vi "New.vi"(8 "error in (no error)":errorcluster, 11 "reference in":refnum<class "[Test Suite] File Transfer Helpers.lvclass">) -> (0 "error out":errorcluster, 3 "reference out":refnum<class "[Test Suite] File Transfer Helpers.lvclass">)   [LabVIEW 2015, in "Tests.lvlib" / "[Test Suite] File Transfer Helpers.lvclass"]
uses:
  [Test Suite] File Transfer Helpers.lvclass
  <vilib>/addons/_JKI Toolkits/VI Tester/TestCase.llb/TestCase.lvclass
  [Test Suite] File Transfer Helpers.lvclass/[Test Suite] File Transfer Helpers.ctl
  <vilib>/addons/_JKI Toolkits/VI Tester/TestSuite.llb/TestSuite.lvclass
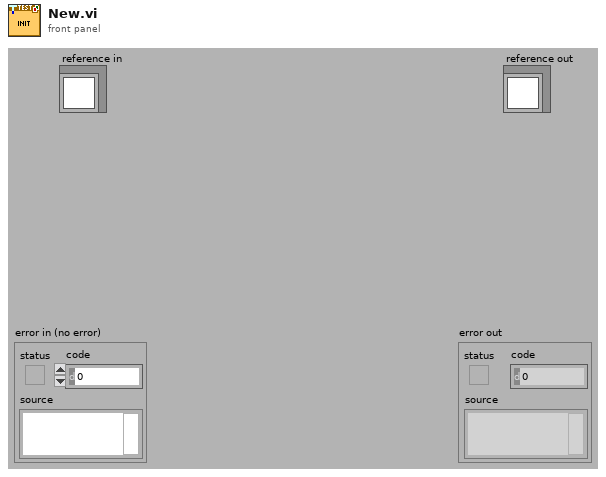
[diagram p1: front panel]
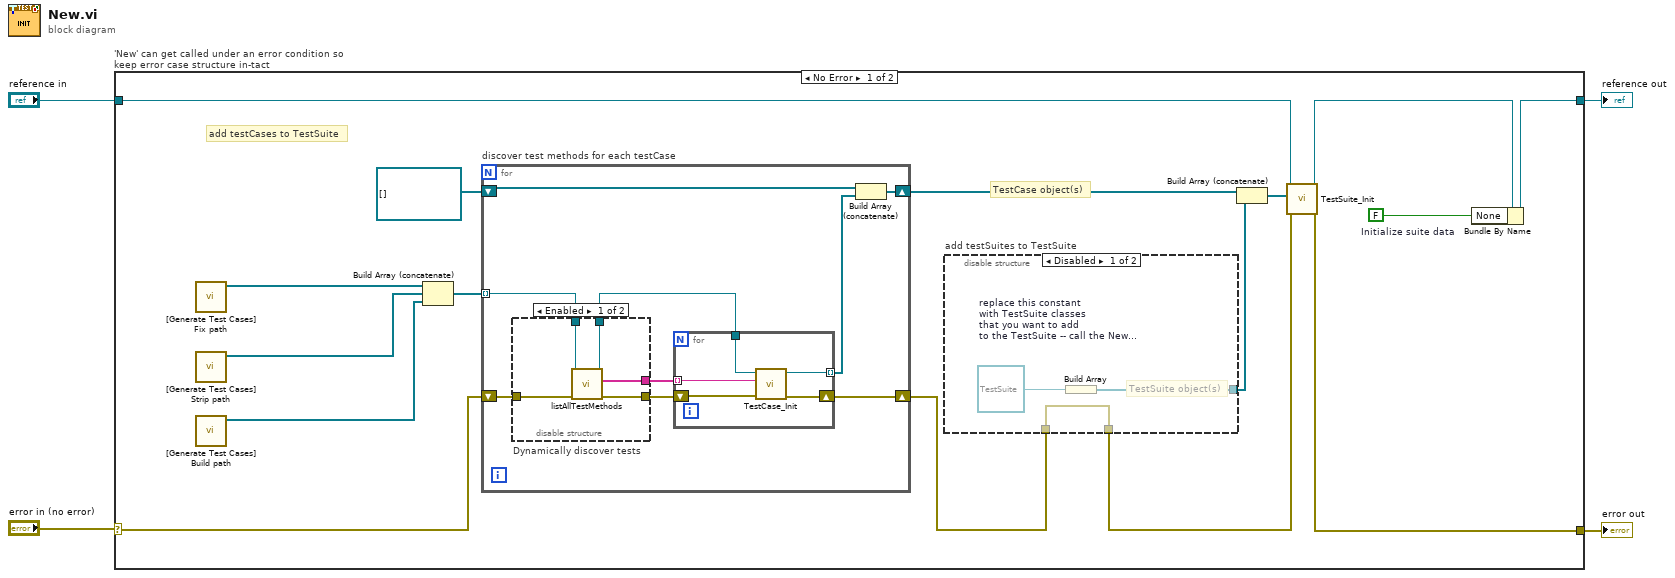
[diagram p0: block diagram]
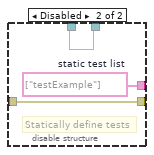
[diagram p2: hidden frame]
diagram:
  n1 = case "'New' can get called under an error condition so keep error case structure in-tact" shown="No Error" "error in (no error)" {
    selector: "error in (no error)" -> [w15 w47]
    tunnel: [w20 w48] -> w4
    tunnel: "reference in" -> [w16 w48]
    tunnel: [w17 w47] -> w1
    frame No Error {
      w19 = FALSE  # Initialize suite data
      # "TestCase object(s)"
      # "add testCases to TestSuite"
      n2 = call "[Generate Test Cases] Fix path.vi"() -> ("Fix Path test cases"=w8:refnum<class "TestCase.lvclass">[])  [unwired: 11 in]
      n3 = call "[Generate Test Cases] Strip path.vi"() -> ("Strip path test cases"=w7:refnum<class "TestCase.lvclass">[])  [unwired: 11 in]
      n4 = call "[Generate Test Cases] Build path.vi"() -> ("Fix Path test cases"=w5:refnum<class "TestCase.lvclass">[])  [unwired: 11 in]
      n5 = Build Array (concatenate)(w8, w7, w5) -> (w6:refnum<class "TestCase.lvclass">[])
      n6 = for "discover test methods for each testCase" {
        shift-right: [w29] -> w10
        shift-left: w15 -> [w25]
        tunnel: w6 -> [w22] mode=indexing
        shift-right: [w26] -> w14
        shift-left: refnum<class "TestCase.lvclass">[] [] -> [w27]
        n7 = disable-structure "Dynamically discover tests" shown="Enabled" {
          disable-tunnel: w25 -> [w34 w35]
          disable-tunnel: [w33 w35] -> w24
          disable-tunnel: [w32 w36] -> w23
          disable-tunnel: w22 -> [w31 w37]
          disable-tunnel: [w30 w37] -> w21
          frame Enabled {
            n8 = call-dynamic "listAllTestMethods.vi"("error in (no error)"=w34, "TestCase in"=w31) -> ("error out"=w33:errorcluster, "test methods"=w32:string[], "TestCase out"=w30:refnum<class "TestCase.lvclass">)  [unwired: 7 in]
          }
          frame Disabled {
            w36 = string[] ["testExample"]  # static test list
            # "Statically define tests"
          }
        }
        n9 = for {
          tunnel: w21 -> [w38]
          tunnel: w23 -> [w42] mode=indexing
          shift-right: [w40] -> w29
          shift-left: w24 -> [w41]
          tunnel: [w39] -> w28 mode=indexing
          n10 = call <vilib>:"TestCase_Init.vi"("error in (no error)"=w41, "methodName (\"runTest\")"=w42, "TestCase in"=w38) -> ("error out"=w40:errorcluster, "TestCase out"=w39:refnum<class "TestCase.lvclass">)  [unwired: 7 in]
        }
        n11 = Build Array (concatenate)(w27, w28) -> (w26:refnum<class "TestCase.lvclass">[])
      }
      n12 = disable-structure "add testSuites to TestSuite" shown="Disabled" {
        disable-tunnel: [w43 _] -> w12
        disable-tunnel: [w45 w46] -> w11
        disable-tunnel: w10 -> [w45 w46]
        frame Disabled {
          w44 = refnum<class "TestSuite.lvclass"> refnum  # replace this constant with TestSuite classes that you want to add to the TestSuite -- call the New method for each TestSuite prior to adding it to this TestSuite
          # "TestSuite object(s)"
          n13 = Build Array(w44) -> (w43:refnum<class "TestSuite.lvclass">[])
        }
        frame Enabled {
          # "by default, no TestSuites are defined\nas members of a TestSuite"
        }
      }
      n14 = Build Array (concatenate)(w14, w12) -> (w13:refnum<class>[])
      n15 = call <vilib>:"TestSuite_Init.vi"("error in (no error)"=w11, "tests (none)"=w13, "TestSuite in"=w16) -> ("error out"=w17:errorcluster, "TestSuite out"=w18:refnum<class "[Test Suite] File Transfer Helpers.lvclass">)  [unwired: 7 in]
      n16 = Bundle By Name(cluster=w18, "None"=w19) -> (w20:refnum<class "[Test Suite] File Transfer Helpers.lvclass">)
    }
    frame Error {
    }
  }
  "reference out" <- w4
  "error out" <- w1
